vi "Switch_feedback_lockin.vi"(8 "error in (no error)":errorcluster, 10 "Z Controller ON/OFF":bool, 11 "Application in":refnum<vi>) -> (0 "error out":errorcluster, 3 "Application out":refnum<vi>)   [LabVIEW 2014]
uses:
  <userlib>/Nanonis Prog Interface V5/Nanonis Prog Interface.lvlib
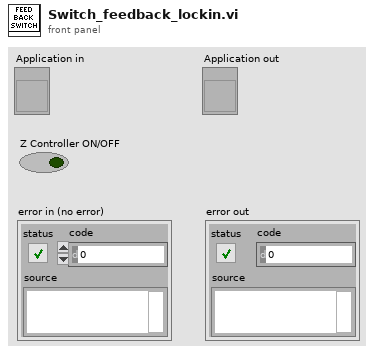
[diagram p1: front panel]
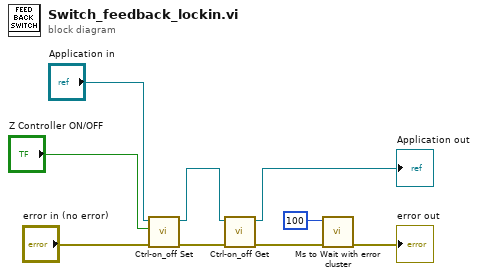
[diagram p0: block diagram]
diagram:
  n1 = call <userlib>:"Ctrl-on_off Set.vi"("error in (no error)"="error in (no error)", "Z Controller ON/OFF"="Z Controller ON/OFF", "Application ref in"="Application in") -> ("error out"=w6:errorcluster, "Application ref out"=w7:refnum<vi>)  [unwired: 7 in]
  n2 = call <userlib>:"Ctrl-on_off Get.vi"("error in (no error)"=w6, "Application ref in"=w7) -> ("error out"=w1:errorcluster, "Application ref out"=→"Application out":refnum<vi>)  [unwired: 7 in, 1 out]
  n3 = call <userlib>:"Ms to Wait with error cluster.vi"("error in (no error)"=w1, "milliseconds to wait"=u32 100) -> ("error out"=→"error out":errorcluster)  [unwired: 4 in, 1 out]
